vi "XmitDisable.vi"(4 "error in (no error)":errorcluster) -> (0 "error out":errorcluster, 1 "Paired = 1":i32, 2 "Switch Verify Sense":string, 3 "Position (0=open, 1=closed)":i32, 6 "Volts Tx Detector Query ShouldBeLow":dbl, 7 "IfTransmittingOne Query ShouldBeNOTx":i32)   [LabVIEW 2009]
doc: "Waveguide switch - H Out - connect to Antenna"
panel:
  # "TBD... Need to include check of TOF power meter"
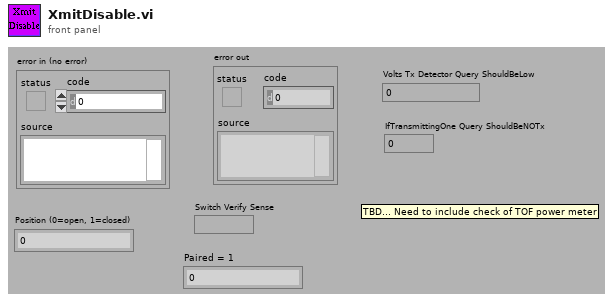
[diagram p1: front panel]
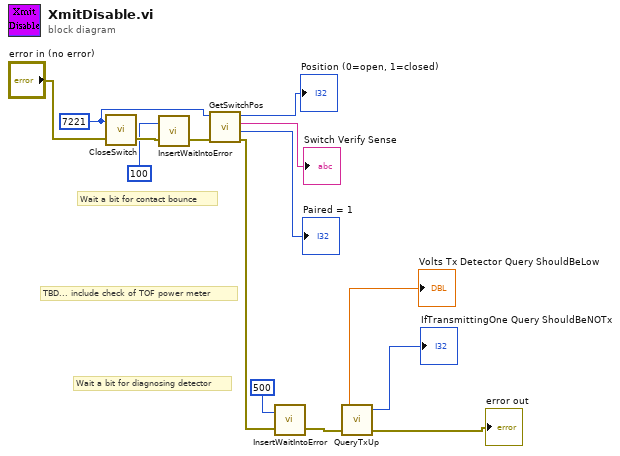
[diagram p0: block diagram]
diagram:
  w13 = 7221
  # "TBD... include check of TOF power meter"
  # "Wait a bit for diagnosing detector"
  # "Wait a bit for contact bounce"
  n1 = call "CloseSwitch.vi"("error in (no error)"="error in (no error)", "Switch ID"=w13) -> ("error out"=w12:errorcluster)  [unwired: 1 in]
  n2 = call "InsertWaitIntoError.vi"("error in (no error)"=w12, "Wait (msecs)"=100) -> ("error out"=w11:errorcluster)  [unwired: 1 in]
  n3 = call "GetSwitchPos.vi"("error in (no error)"=w11, "Circuit ID"=w13) -> ("Error out"=w6:errorcluster, "Paired = 1"=→"Paired = 1":i32, "Switch Position Verify  Sense"=→"Switch Verify Sense":string, "Position (0=open, 1=closed)"=→"Position (0=open, 1=closed)":i32)  [unwired: 2 in]
  n4 = call "InsertWaitIntoError.vi"("error in (no error)"=w6, "Wait (msecs)"=500) -> ("error out"=w5:errorcluster)  [unwired: 1 in]
  n5 = call "QueryTxUp.vi"("error in (no error)"=w5) -> ("error out"=→"error out":errorcluster, "IfTransmittingOne"=→"IfTransmittingOne Query ShouldBeNOTx":i32, "Volts Tx Detector"=→"Volts Tx Detector Query ShouldBeLow":dbl)  [unwired: 1 in, 1 out]
